vi "multiply.vi"() -> ()   [LabVIEW 2022 SP3]
uses:
  <vilib>/Utility/error.llb/DialogType.ctl
panel:
  in  "val_int2":i32=3
  out "return val":i32
  out "error":string
  out "error out":errorcluster
  in  "val_int":i32=10
  in  "Python version":string="3.9"
  in  "module path":path=path "R:/work/LabVIEW-and-Python-interop/interop/interop.py"
  in  "error in":errorcluster
  in  "Python path":path=path "C:/Users/Mikio Fukushima/AppData/Local/Programs/Python/Python39/python.exe"
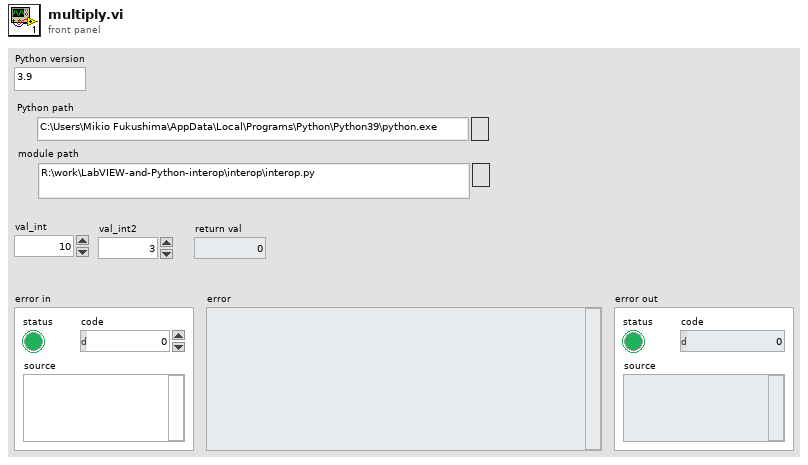
[diagram p1: front panel]
types:
  T1 = typedef "DialogType.ctl" = u16
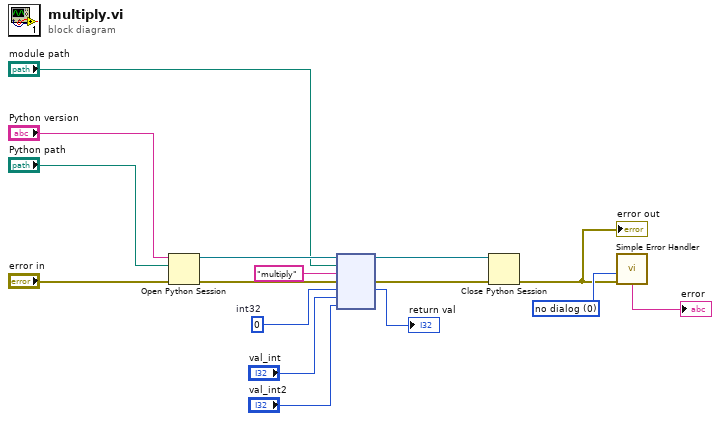
[diagram p0: block diagram]
diagram:
  w4 = 0  # int32
  w8 = T1 0 items=["no dialog", "OK message", "continue or stop message", "OK message + warnings", "continue/stop + warnings"] ("type of dialog (OK msg:1)")
  n1 = Open Python Session(python version="Python version", python path="Python path", 3:"error in") -> (session out=w15:refnum<k35>, error out=w2:errorcluster)
  n2 = node(w15, "module path", "multiply" ("function name"), w2, w4, "val_int", "val_int2") -> (w6:refnum<k35>, w1:errorcluster, →"return val":i32)  [unwired: 2 in, 2 out]
  n3 = Close Python Session(session in=w6, error in=w1) -> (11:w7:errorcluster)
  "error out" <- w7
  n4 = call <vilib>:"Simple Error Handler.vi"("type of dialog (OK msg:1)"=w8, "error in (no error)"=w7) -> ("message"=→"error":string)  [unwired: 3 in, 4 out]
